vi "Subvi Valid US Phone.vi"(0 "PhNumString":string) -> (1 "Is Valid":bool, 2 "Valid Number":string)   [LabVIEW 2012]
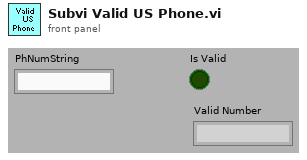
[diagram p1: front panel]
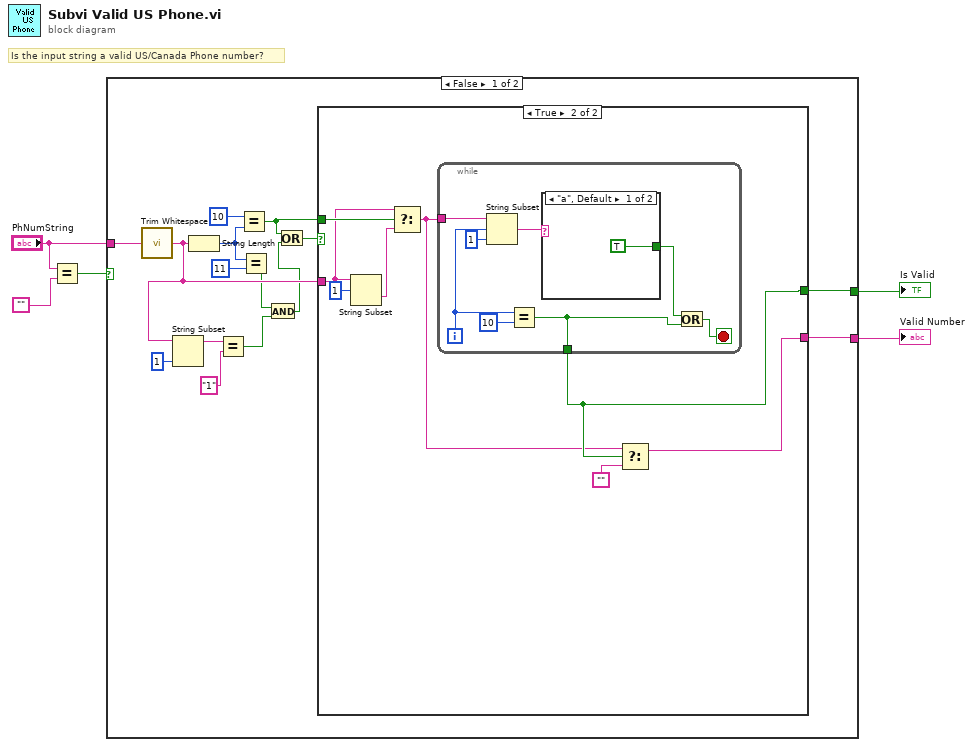
[diagram p0: block diagram]
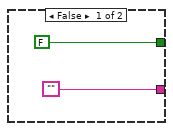
[diagram p2: hidden frame]
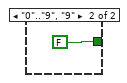
[diagram p3: hidden frame]
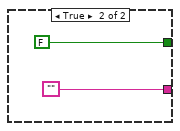
[diagram p4: hidden frame]
diagram:
  # "Is the input string a valid US/Canada Phone number?"
  n1 = Equal?(x="PhNumString", y="") -> (x = y?=w4:bool)
  n2 = case shown="False" w4 {
    tunnel: [w15 FALSE] -> w3
    tunnel: [w14 ""] -> w2
    tunnel: "PhNumString" -> [w20 _]
    frame False {
      n3 = call <vilib>:"Trim Whitespace.vi"("string"=w20) -> ("trimmed string"=w10:string)  [unwired: 1 in]
      n4 = String Subset(string=w10, length (rest)=1 ("length (rest)")) -> (substring=w12:string)  [unwired: 1 out]
      n5 = String Length(string=w10) -> (length=w18:i32)
      n6 = Equal?(x=w12, y="1") -> (x = y?=w8:bool)
      n7 = Equal?(x=10, y=w18) -> (x = y?=w6:bool)
      n8 = Equal?(x=w18, y=11) -> (x = y?=w9:bool)
      n9 = And(x=w9, y=w8) -> (x .and. y?=w7:bool)
      n10 = Or(x=w6, y=w7) -> (x .or. y?=w16:bool)
      n11 = case shown="True" w16 {
        tunnel: [FALSE w25] -> w15
        tunnel: ["" w26] -> w14
        tunnel: w10 -> [_ w28]
        tunnel: w6 -> [_ w30]
        frame False {
        }
        frame True {
          n12 = String Subset(string=w28, offset (0)=1) -> (substring=w24:string)  [unwired: 1 out]
          n13 = Select(t=w28, s=w30, f=w24) -> (s? t:f=w23:string)
          n14 = while {
            tunnel: w23 -> [w38]
            tunnel: [w31] -> w25
            i -> [w35]
            stop <- w33 stop-if-true
            n15 = String Subset(string=w38, offset (0)=w35, length (rest)=1 ("length (rest)")) -> (substring=w36:string)
            n16 = Equal?(x=w35, y=10) -> (x = y?=w31:bool)
            n17 = case shown="\"a\", Default" w36 {
              tunnel: [TRUE FALSE] -> w32
              frame "a", Default {
              }
              frame "0".."9", "9" {
              }
            }
            n18 = Or(x=w32, y=w31) -> (x .or. y?=w33:bool)
          }
          n19 = Select(t=w23, s=w25, f="") -> (s? t:f=w26:string)
        }
      }
    }
    frame True {
    }
  }
  "Is Valid" <- w3
  "Valid Number" <- w2
